vi "MCLB Request Edit Cell.vi"(8 "error in (no error)":errorcluster, 10 "Cell Position":T1, 11 "View in":refnum<class "RTM View.lvclass">) -> (0 "error out":errorcluster, 1 "Edited Cell":T1, 2 "Value":string, 3 "View out":refnum<class "RTM View.lvclass">, 5 "Modified?":bool)   [LabVIEW 2013, in "SET Project Editor.lvlib" / "RTM View.lvclass"]
uses:
  RTM View.lvclass
  <vilib>/Utility/miscctls.llb/LVRowAndColumnTypeDef.ctl
  MCListbox View/MCListbox View.lvclass
  RTM View.lvclass/RTM View.ctl
  <vilib>/ActorFramework/Actor/Actor.lvclass/Actor.ctl
  <vilib>/ActorFramework/Message Enqueuer/Message Enqueuer.lvclass/Message Enqueuer.ctl
  <vilib>/ActorFramework/Message Enqueuer/Enqueue.vi
  <vilib>/ActorFramework/Message Priority Queue/Priority Enqueue.vi
  Controller Messages/Set Modified Flag Msg/Set Modified Flag Msg.lvclass
  <vilib>/ActorFramework/Actor/Actor.lvclass
  SET Project Data/Menu Class/Menu Data.lvclass
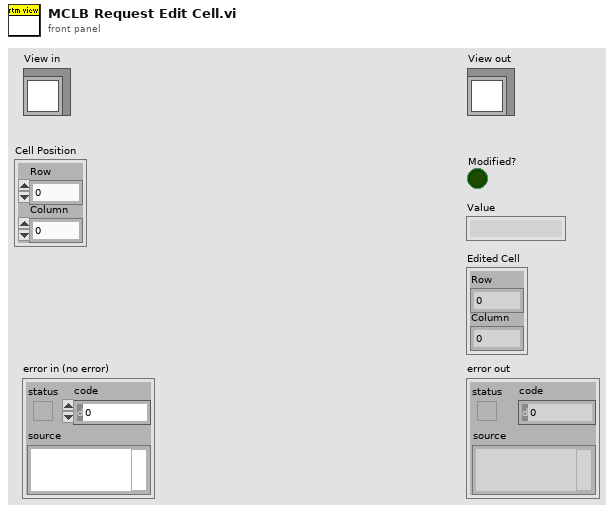
[diagram p1: front panel]
types:
  T1 = typedef "LVRowAndColumnTypeDef.ctl" = cluster{"Row":i32, "Column":i32}
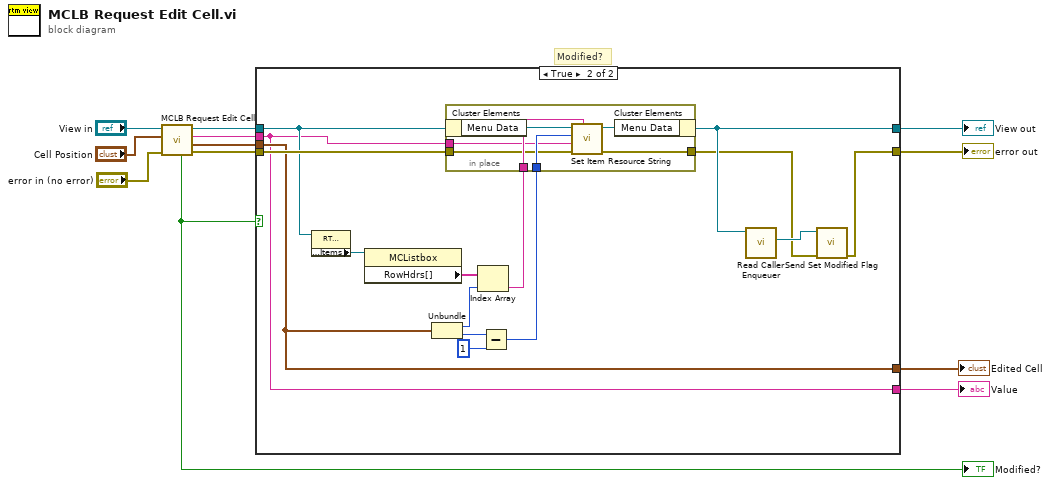
[diagram p0: block diagram]
diagram:
  # "Modified?"
  n1 = call-parent "MCLB Request Edit Cell.vi"("error in (no error)"="error in (no error)", "RowAndCollumn"="Cell Position", "View in"="View in") -> ("error out"=w9:errorcluster, "Edited Cell"=w6:T1, "Value"=w8:string, "View out"=w7:refnum<class "RTM View.lvclass">, "Modified?"=w1:bool)  [unwired: 4 in]
  "Modified?" <- w1
  n2 = case shown="True" w1 {
    tunnel: w9 -> [w15 w31]
    tunnel: w8 -> [w14 w17]
    tunnel: w7 -> [w16 w26]
    tunnel: w6 -> [w13 w18]
    tunnel: [w15 w20] -> w5
    tunnel: [w16 w21] -> w4
    tunnel: [w13 w18] -> w3
    tunnel: [w14 w17] -> w2
    frame False {
    }
    frame True {
      n3 = property class="RTM View.lvclass"(reference=w26) -> ("Properties:Items"=w25:refnum<vi>)  [unwired: 1 in, 2 out]
      n4 = property class="MCListbox"(reference=w25) -> ("RowHdrs[]"=w27:string[])  [unwired: 1 in, 2 out]
      n5 = Unbundle(w18) -> ("Row"=w28:i32, "Column"=w29:i32)
      n6 = Index Array(array=w27, index=w28) -> (element=w24:string)
      n7 = Subtract(x=w29, y=1) -> (x-y=w23:i32)
      n8 = in-place {
        in-place-border: w24 -> [w37]
        in-place-border: w17 -> [w35]
        in-place-border: w23 -> [w36]
        in-place-border: w31 -> [w33]
        in-place-border: [w32] -> w19
        n9 = in-place-cluster #1(w26) -> ("Menu Data"=w38:refnum<class "Menu Data.lvclass">)
        n10 = call "Set Item Resource String.vi"("ItemName (ASCII)"=w37, "error in (no error)"=w33, "Text (UTF-16)"=w35, "Language"=w36, "Menu Data in"=w38) -> ("error out"=w32:errorcluster, "Menu Data out"=w34:refnum<class "Menu Data.lvclass">)  [unwired: 5 in]
        n11 = in-place-cluster #1("Menu Data"=w34) -> (w21:refnum<class "RTM View.lvclass">)
      }
      n12 = call <vilib>:"Read Caller Enqueuer.vi"("Actor"=w21) -> ("Caller Enqueuer"=w22:refnum<class "Message Enqueuer.lvclass">)  [unwired: 10 in]
      n13 = call "Send Set Modified Flag.vi"("error in (no error)"=w19, "Message Enqueuer"=w22) -> ("error out"=w20:errorcluster)  [unwired: 8 in, 1 out]
    }
  }
  "error out" <- w5
  "View out" <- w4
  "Value" <- w2
  "Edited Cell" <- w3
